vi "Sort Fast Tree Structure Geo and Ref.vi"(10 "Node":T2, 11 "Tree":T1(array[cluster])) -> (2 "Geometric Items":T1(array[cluster]), 3 "Reference Items":T1(array[cluster]))   [LabVIEW 2019, in "ParseGDSII.lvclass"]
uses:
  ParseGDSII.lvclass
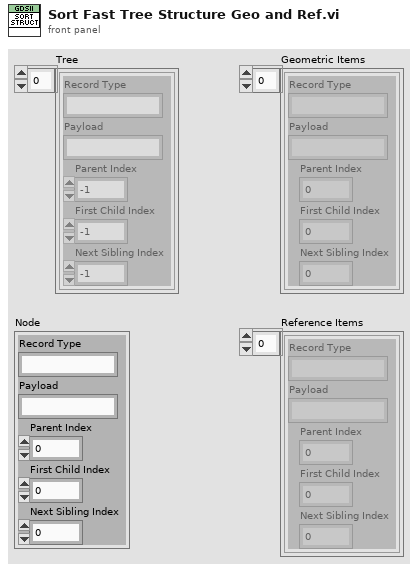
[diagram p1: front panel]
types:
  T1 = cluster{"Record Type":string, "Payload":string, "Parent Index":i32, "First Child Index":i32, "Next Sibling Index":i32}[]
  T2 = cluster{"Record Type":string, "Payload":string, "Parent Index":i32, "First Child Index":i32, "Next Sibling Index":i32}
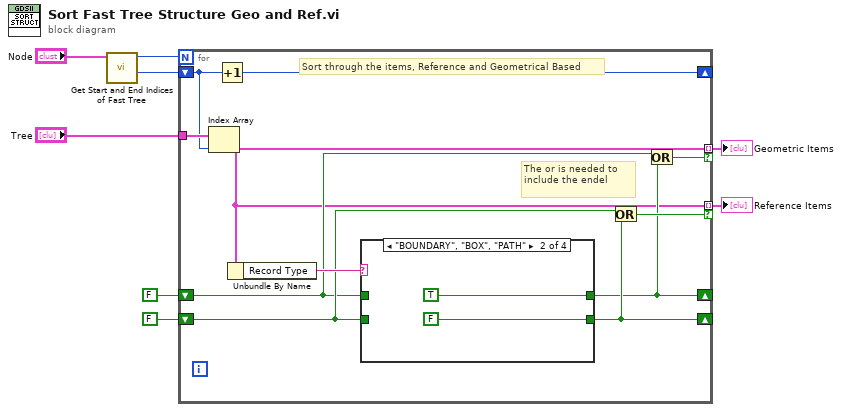
[diagram p0: block diagram]
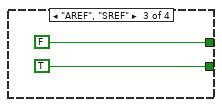
[diagram p3: hidden frame]
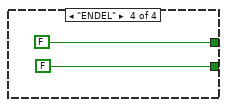
[diagram p4: hidden frame]
diagram:
  n1 = call "Get Start and End Indices of Fast Tree.vi"("Node"="Node") -> ("Index"=w1:i32, "Length"=w2:i32)  [unwired: 9 in]
  n2 = for {
    N: w2 -> [_]
    shift-right: [w12] -> _
    shift-left: FALSE -> [w10]
    tunnel: [w9] -> w5 mode=indexing if=w11
    tunnel: "Tree" -> [w18]
    shift-right: [w16] -> _
    shift-left: w1 -> [w17]
    shift-right: [w15] -> _
    shift-left: FALSE -> [w14]
    tunnel: [w9] -> w4 mode=indexing if=w13
    # "The or is needed to include the endel"
    # "Sort through the items, Reference and Geometrical Based"
    n3 = Index Array(array=w18, index=w17) -> (element=w9:T2)
    n4 = Increment(x=w17) -> (x+1=w16:i32)
    n5 = Unbundle By Name(w9) -> ("Record Type"=w19:string)
    n6 = case shown="\"BOUNDARY\", \"BOX\", \"PATH\"" w19 {
      tunnel: [w21 TRUE FALSE FALSE] -> w12
      tunnel: w10 -> [w21 _ _ _]
      tunnel: [w20 FALSE TRUE FALSE] -> w15
      tunnel: w14 -> [w20 _ _ _]
      frame Default {
      }
      frame "BOUNDARY", "BOX", "PATH" {
      }
      frame "AREF", "SREF" {
      }
      frame "ENDEL" {
      }
    }
    n7 = Or(x=w14, y=w15) -> (x .or. y?=w13:bool)
    n8 = Or(x=w10, y=w12) -> (x .or. y?=w11:bool)
  }
  "Geometric Items" <- w5
  "Reference Items" <- w4
